vi "Asana Oauth.vi"(6 "error in (no error)":errorcluster, 9 "Auth Time In":dbl) -> (0 "error out":errorcluster, 1 "Path":path, 2 "Codes":T1, 3 "Auth Time Out":dbl)   [LabVIEW 2016]
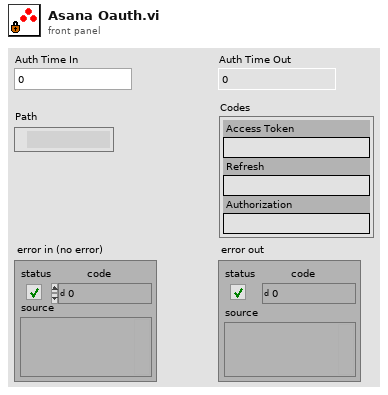
[diagram p1: front panel]
types:
  T1 = cluster{"Access Token":string, "Refresh":string, "Authorization":string}
  T2 = cluster{"Access":string, "Refresh":string, "Authorization":string}
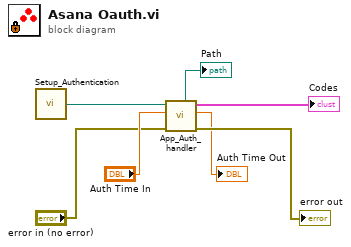
[diagram p0: block diagram]
diagram:
  n1 = call "Setup_Authentication.vi"() -> ("file path"=w4:path)  [unwired: 1 in]
  n2 = call "App_Auth_handler.vi"("error in (no error)"="error in (no error)", "Auth Time In"="Auth Time In", "Path In"=w4) -> ("error out"=→"error out":errorcluster, "Auth Time Out"=→"Auth Time Out":dbl, "Cluster"=→"Codes":T2, "Path Out"=→"Path":path)  [unwired: 5 in]
